vi "_wmg_readItems2.vi"(2 "input_p":i32[](array[numeric]), 3 "input":string[](array[string]), 4 "input_sp":string[](array[string])) -> (0 "output_p":i32[](array[numeric]), 1 "output_sp":string[](array[string]))   [LabVIEW 2011]
panel:
  in  "列表框":i32(listbox)
  out "数组 2":i32[](array[numeric])
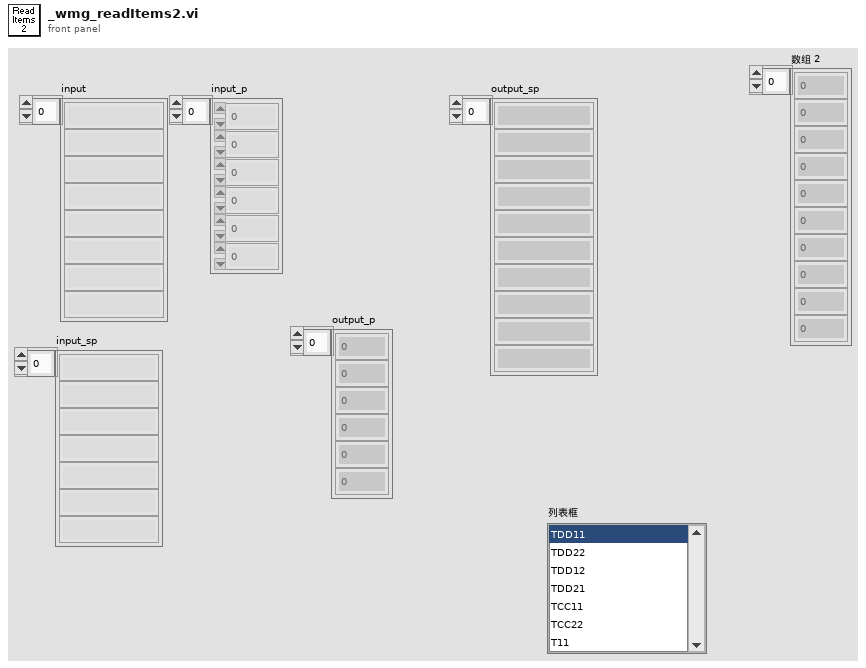
[diagram p1: front panel]
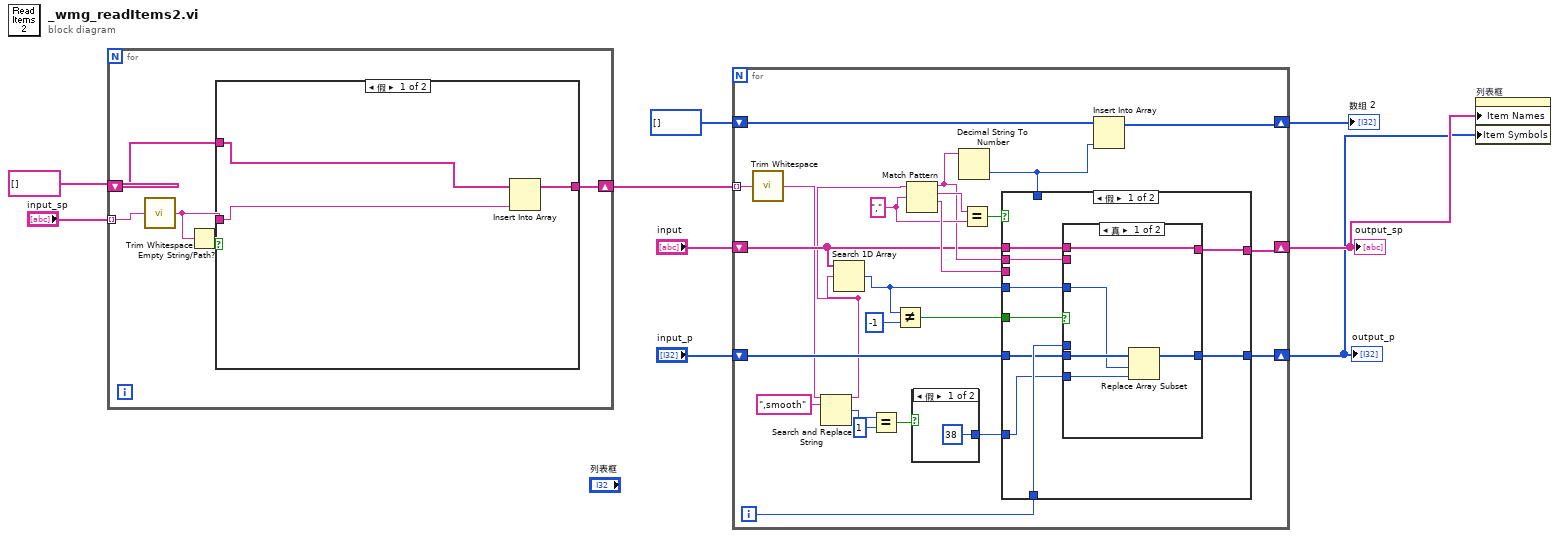
[diagram p0: block diagram]
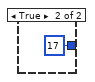
[diagram p3: hidden frame]
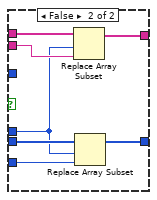
[diagram p4: hidden frame]
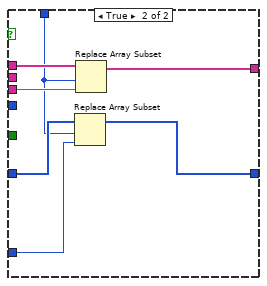
[diagram p5: hidden frame]
diagram:
  n1 = for {
    tunnel: "input_sp" -> [w14] mode=indexing
    shift-right: [w11] -> w5
    shift-left: string[] [] -> [w12]
    n2 = call <vilib>:"Trim Whitespace.vi"("string"=w14) -> ("trimmed string"=w10:string)  [unwired: 1 in]
    n3 = Empty String/Path?(string/path=w10) -> (empty?=w13:bool)
    n4 = case shown="假" w13 {
      tunnel: w12 -> [w17 w18]
      tunnel: [w16 w18] -> w11
      tunnel: w10 -> [w15 _]
      frame False {
        n5 = Insert Into Array(array=w17, new element=w15) -> (w16:string[])  [unwired: 1 in]
      }
      frame True {
      }
    }
  }
  n6 = for {
    tunnel: w5 -> [w42] mode=indexing
    shift-right: [w40] -> w2
    shift-left: "input" -> [w29]
    shift-right: [w38] -> w1
    shift-left: "input_p" -> [w39]
    shift-right: [w35] -> w3
    shift-left: i32[] [] -> [w37]
    i -> [w30]
    w33 = "," ("正则表达式")
    n7 = call <vilib>:"Trim Whitespace.vi"("string"=w42) -> ("trimmed string"=w25:string)  [unwired: 1 in]
    n8 = Search and Replace String(input string=w25, search string=",smooth" ("搜索字符串")) -> (result string=w19:string, number of replacements=w23:i32)  [unwired: 6 in, 2 out]
    n9 = Search 1D Array(1D array=w29, element=w19) -> (index of element=w28:i32)  [unwired: 1 in]
    n10 = Equal?(x=w23, y=1) -> (x = y?=w21:bool)
    n11 = Not Equal?(x=w28, y=-1) -> (x != y?=w26:bool)
    n12 = Match Pattern(string=w19, regular expression=w33) -> (before substring=w31:string, match substring=w34:string, after substring=w41:string)  [unwired: 1 in, 1 out]
    n13 = case shown="假" w21 {
      tunnel: [38 17] -> w20
      frame False {
      }
      frame True {
      }
    }
    n14 = Decimal String To Number(string=w31) -> (number=w36:i32)  [unwired: 2 in, 1 out]
    n15 = Equal?(x=w34, y=w33) -> (x = y?=w32:bool)
    n16 = case shown="假" w32 {
      tunnel: w29 -> [w53 w72]
      tunnel: w41 -> [_ w71]
      tunnel: [w50 w70] -> w40
      tunnel: w39 -> [w49 w69]
      tunnel: [w48 w68] -> w38
      tunnel: w36 -> [_ w67]
      tunnel: w31 -> [w52 _]
      tunnel: w30 -> [w51 _]
      tunnel: w28 -> [w47 _]
      tunnel: w26 -> [w46 _]
      tunnel: w20 -> [w45 w66]
      frame False {
        n17 = case shown="真" w46 {
          tunnel: w53 -> [w55 w65]
          tunnel: w52 -> [_ w64]
          tunnel: w51 -> [_ w60]
          tunnel: [w55 w63] -> w50
          tunnel: w49 -> [w58 w62]
          tunnel: [w57 w61] -> w48
          tunnel: w47 -> [w56 _]
          tunnel: w45 -> [w54 w59]
          frame True {
            n18 = Replace Array Subset(array=w58, new element=w54, index=w56) -> (w57:i32[])
          }
          frame False {
            n19 = Replace Array Subset(array=w65, new element=w64, index=w60) -> (w63:string[])
            n20 = Replace Array Subset(array=w62, new element=w59, index=w60) -> (w61:i32[])
          }
        }
      }
      frame True {
        n21 = Replace Array Subset(array=w69, new element=w66, index=w67) -> (w68:i32[])
        n22 = Replace Array Subset(array=w72, new element=w71, index=w67) -> (w70:string[])
      }
    }
    n23 = Insert Into Array(array=w37, new element=w36) -> (w35:i32[])  [unwired: 1 in]
  }
  "output_sp" <- w2
  "output_p" <- w1
  "数组 2" <- w3
  n24 = property on="列表框" class="LstBox (严格)"("Item Names"=w2, "Item Symbols"=w1) -> ()  [unwired: 2 in, 2 out]
